vi "SetVelocityConfig.vi"(8 "error in (no error)":errorcluster, 11 "KST101 in":refnum<class "KST101.lvclass">) -> (0 "error out":errorcluster, 3 "KST101 out":refnum<class "KST101.lvclass">)   [LabVIEW 2016, in "Stepper Motor Controller.lvlib" / "KST101.lvclass"]
uses:
  KST101.lvclass
  KST101.lvclass/KST101.ctl
  D:/Workspace/ProCyteOne_LaserModuleAlignment/shared/Thorlabs/Kinesis/Dependencies/Thorlabs.MotionControl.KCube.StepperMotorCLI.dll
  Dependencies/Thorlabs.MotionControl.KCube.StepperMotorCLI.dll
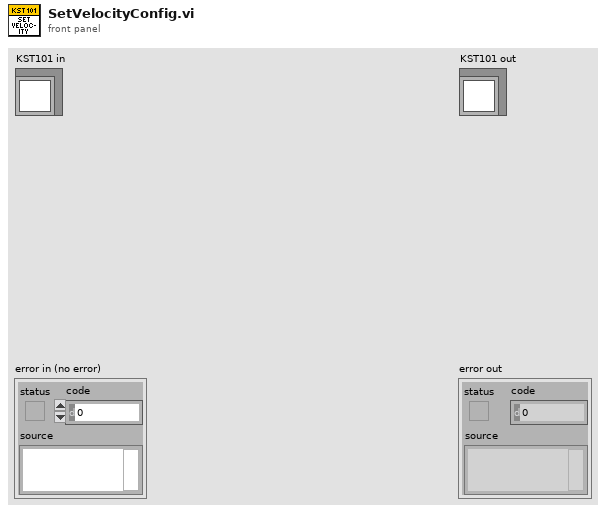
[diagram p1: front panel]
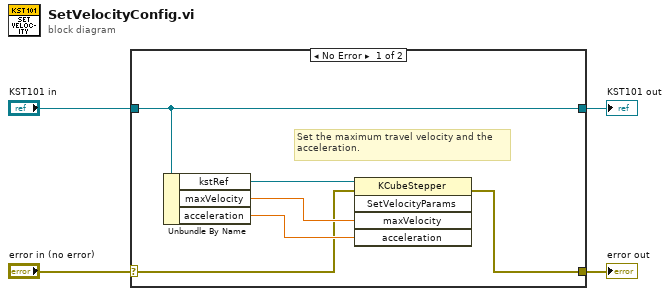
[diagram p0: block diagram]
diagram:
  n1 = case shown="No Error" "error in (no error)" {
    selector: "error in (no error)" -> [w6 w12]
    tunnel: [w5 w12] -> w3
    tunnel: [w10 w11] -> w1
    tunnel: "KST101 in" -> [w10 w11]
    frame No Error {
      # "Set the maximum travel velocity and the\nacceleration."
      n2 = Unbundle By Name(w10) -> ("kstRef"=w9:refnum<k24>, "maxVelocity"=w8:dbl, "acceleration"=w7:dbl)
      n3 = invoke class="KCubeStepper" method="SetVelocityParams"(reference=w9, error in=w6, "maxVelocity"=w8, "acceleration"=w7) -> (error out=w5:errorcluster)  [unwired: 1 in, 4 out]
    }
    frame Error {
    }
  }
  "error out" <- w3
  "KST101 out" <- w1
